vi "Test Oscillator f.vi"(8 "error in (no error)":errorcluster, 11 "VISA resource name":refnum<visa-resource-name>) -> (0 "error out":errorcluster, 3 "VISA resource name":refnum<visa-resource-name>)   [LabVIEW 2019, in "SR7270 Drivers.lvlib"]
uses:
  SR7270 Drivers.lvlib
  <userlib>/_OpenG.lib/numeric/numeric.llb/Random Number Within Range - DBL__ogtk.vi
  <vilib>/addons/_JKI Toolkits/Caraya/classes/Test/Test.lvclass
  <vilib>/addons/_JKI Toolkits/Caraya/classes/Assert/Assert.lvclass
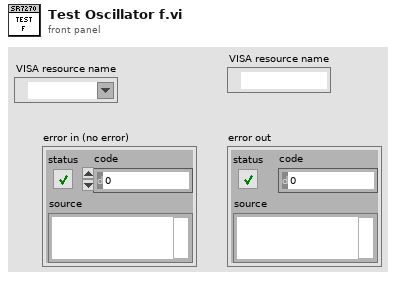
[diagram p1: front panel]
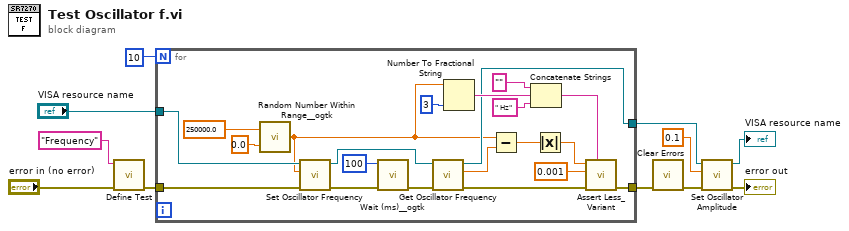
[diagram p0: block diagram]
diagram:
  n1 = call <vilib>:"Define Test.vi"("error in (no error)"="error in (no error)", "Label (VI Title)"="Frequency") -> ("error out"=w7:errorcluster)  [unwired: 9 in]
  n2 = for {
    N: 10 -> [_]
    tunnel: "VISA resource name" -> [w18]
    tunnel: w7 -> [w24]
    tunnel: [w19] -> w11
    tunnel: [w16] -> w4
    n3 = call-poly <userlib>:"Random Number Within Range__ogtk.vi"("High"=250000.0, "Low"=0.0) -> ("Random Number"=w15:dbl)  [unwired: 3 in]
    n4 = call "Set Oscillator Frequency.vi"("error in (no error)"=w24, "Oscillator Frequency (Hz)"=w15, "VISA resource name"=w18) -> ("error out"=w23:errorcluster, "VISA resource name out"=w17:refnum<visa-resource-name>)  [unwired: 7 in]
    n5 = call <userlib>:"Wait (ms)__ogtk.vi"("error in (no error)"=w23, "milliseconds to wait"=u32 100) -> ("error out"=w22:errorcluster)  [unwired: 8 in, 1 out]
    n6 = call "Get Oscillator Frequency.vi"("error in (no error)"=w22, "VISA resource name"=w17) -> ("error out"=w21:errorcluster, "Oscillator Frequency (Hz)"=w20:dbl, "VISA resource name out"=w16:refnum<visa-resource-name>)  [unwired: 7 in]
    n7 = Number To Fractional String(number=w15, precision (6)=i16 3) -> (F-format string=w29:string)  [unwired: 2 in]
    n8 = Subtract(x=w15, y=w20) -> (x-y=w25:dbl)
    n9 = Concatenate Strings("" ("string"), w29, " Hz" ("string")) -> (w13:string)
    n10 = Absolute Value(x=w25) -> (abs(x)=w26:dbl)
    n11 = call <vilib>:"Assert Less_Variant.vi"("Label"=w13, "error in (no error)"=w21, "Y"=0.001 ("Phase (°)"), "X"=w26) -> ("error out"=w19:errorcluster)  [unwired: 7 in]
  }
  n12 = call <vilib>:"Clear Errors.vi"("error in (no error)"=w11) -> ("error out"=w6:errorcluster)  [unwired: 5 in, 1 out]
  n13 = call "Set Oscillator Amplitude.vi"("error in (no error)"=w6, "Oscillator Amplitude (V)"=0.1, "VISA resource name"=w4) -> ("error out"=→"error out":errorcluster, "VISA resource name out"=→"VISA resource name":refnum<visa-resource-name>)  [unwired: 7 in]
